vi "WriteDB.vi"(1 "NG?":bool, 4 "曲线数组":refnum<vi>[](array[refnum])) -> ()   [LabVIEW 2018]
uses:
  <vilib>/addons/database/Connection.llb/DB Tools Open Connec (Path).vi
  <vilib>/addons/database/NI_Database_API.lvlib
panel:
  in  "停止":bool
  out "上传状态":string
  in  "SQL_Data":T1={"cMacCode"="1-C-229", "cInvCode"="F100151288", "cCheckDate"="2018-10-31 13:02:50", "cCheckNo"="00013", "cState"="OK", "cDefine1"="OK", "cDefine2"="OK", "cDefine3"="OK", "cDefine4"="OK", "cDefine5"="OK", "cDefine6"="OK", "cDefine7"="8.78", "cDefine8"="6.96", "cDefine9"="2.24", "cDefine10"="1.64", "cDefine11"="1.74", "cDefine12"="+0.54", "cDefine13"="1.48", "cDefine14"="1.47", "cDefine15"="2.07", "cDefine16"="+0.51", "cDefine17"="0", "cDefine18"="0", "cDefine20"="0", "cDefine19"="0", "cDefine21"="0", "cDefine22"="0", "cDefine23"="0", "cDefine24"="0", "cDefine25"="0", "cDefine26"="0", "cDefine27"="0", "cDefine28"="0", "cDefine29"="0", "cDefine30"="0", "cDefine31"="0", "cDefine32"="0", "cDefine33"="0", "cDefine34"="0", "cDefine35"="0", "cDefine36"="0", "cDefine37"="0", "cDefine38"="0", "cDefine39"="0", "cDefine40"="0", "cDefine41"="0", "cDefine42"="0", "cDefine43"="0", "cDefine44"="0", "cDefine45"="0", "cDefine46"="0", "cDefine47"="0", "cDefine48"="0"} caption="上传数据"
  out "error out":errorcluster caption="错误信息" {"code" format="%.0x"}
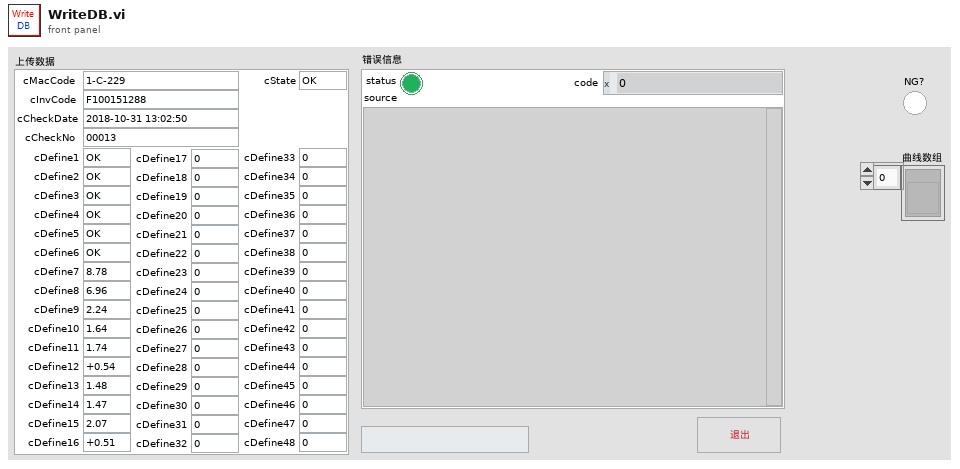
[diagram p1: front panel]
types:
  T1 = cluster{"cMacCode":string, "cInvCode":string, "cCheckDate":string, "cCheckNo":string, "cState":string, "cDefine1":string, "cDefine2":string, "cDefine3":string, "cDefine4":string, "cDefine5":string, "cDefine6":string, "cDefine7":string, "cDefine8":string, "cDefine9":string, "cDefine10":string, "cDefine11":string, "cDefine12":string, "cDefine13":string, "cDefine14":string, "cDefine15":string, "cDefine16":string, "cDefine17":string, "cDefine18":string, "cDefine20":string, "cDefine19":string, "cDefine21":string, "cDefine22":string, "cDefine23":string, "cDefine24":string, "cDefine25":string, "cDefine26":string, "cDefine27":string, "cDefine28":string, "cDefine29":string, "cDefine30":string, "cDefine31":string, "cDefine32":string, "cDefine33":string, "cDefine34":string, "cDefine35":string, "cDefine36":string, "cDefine37":string, "cDefine38":string, "cDefine39":string, "cDefine40":string, "cDefine41":string, "cDefine42":string, "cDefine43":string, "cDefine44":string, "cDefine45":string, "cDefine46":string, "cDefine47":string, "cDefine48":string}
  T2 = typedef "NI_Database_API.lvlib/Conn ObjectReference.ctl" = refnum<k1>
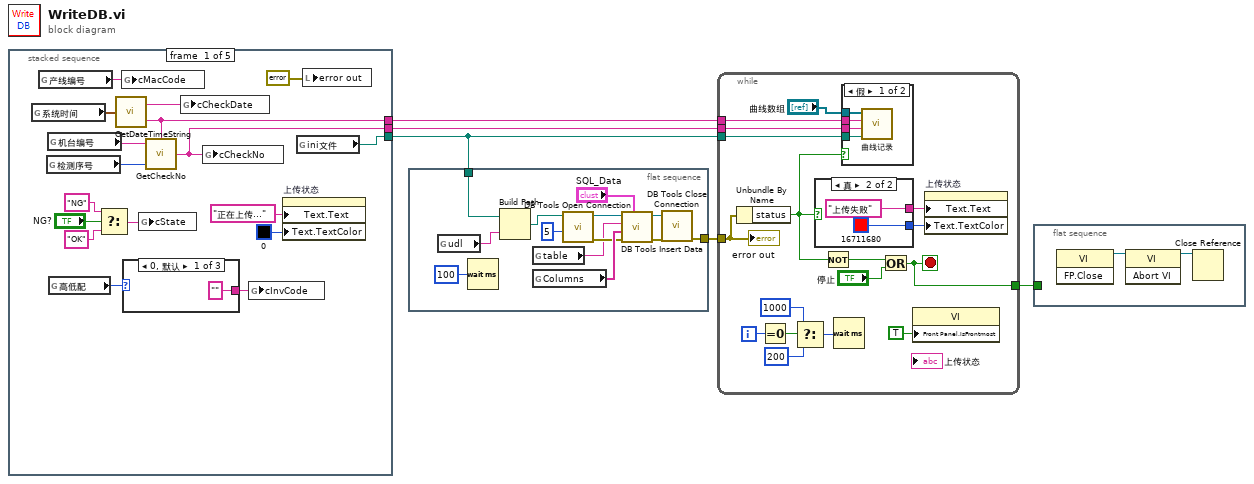
[diagram p0: block diagram]
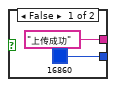
[diagram p3: hidden frame]
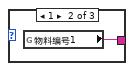
[diagram p4: hidden frame]
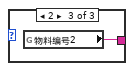
[diagram p5: hidden frame]
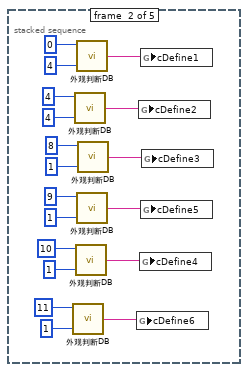
[diagram p6: hidden frame]
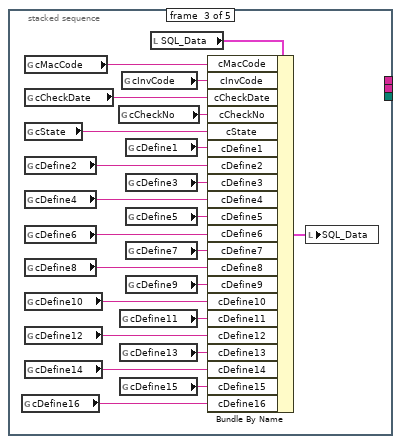
[diagram p7: hidden frame]
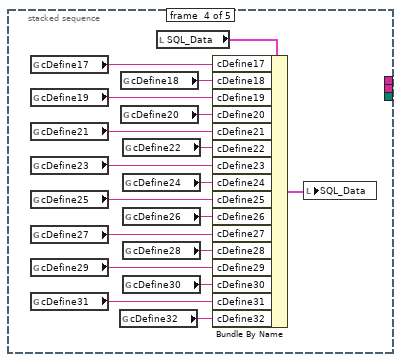
[diagram p8: hidden frame]
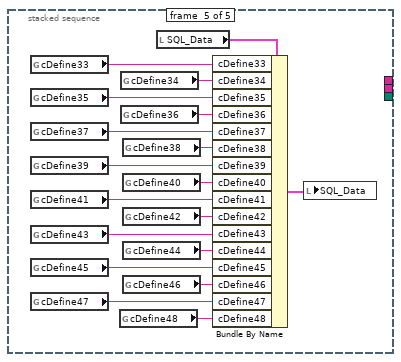
[diagram p9: hidden frame]
diagram:
  n1 = stacked-sequence {
    tunnel: [w8 _ _ _ _] -> w2
    tunnel: [w7 _ _ _ _] -> w3
    tunnel: [w6 _ _ _ _] -> w1
    frame #0 {
      n2 = global read "全局 1.vi" "系统时间"() -> (w9:timestamp)
      n3 = global read "全局 1.vi" "产线编号"() -> (w20:string)
      n4 = global read "全局 1.vi" "检测序号"() -> (w17:u16)
      n5 = global read "全局 1.vi" "机台编号"() -> (w18:string)
      n6 = global read "全局 1.vi" "高低配"() -> (w22:i16)
      n7 = Select(t="NG", s="NG?", f="OK") -> (s? t:f=w12:string)
      n8 = call "GetDateTimeString.vi"("time stamp"=w9) -> ("YYYYMMDD"=w7:string, "date/time string"=w19:string)  [unwired: 3 in]
      n9 = global write "全局SQL.vi" "cMacCode"(w20) -> ()
      n10 = case shown="0, 默认" w22 {
        tunnel: ["" ("物料编号2") w24 w25] -> w21
        frame 0, Default {
        }
        frame 1 {
          n11 = global read "全局 1.vi" "物料编号1"() -> (w24:string)
        }
        frame 2 {
          n12 = global read "全局 1.vi" "物料编号2"() -> (w25:string)
        }
      }
      n13 = global write "全局SQL.vi" "cState"(w12) -> ()
      n14 = call "GetCheckNo.vi"("年月日"=w7, "序号"=w17, "机台编号"=w18) -> ("CheckNo"=w8:string)  [unwired: 1 in]
      n15 = global write "全局SQL.vi" "cCheckDate"(w19) -> ()
      n16 = global write "全局SQL.vi" "cCheckNo"(w8) -> ()
      n17 = global write "全局SQL.vi" "cInvCode"(w21) -> ()
      n18 = property on="上传状态" class="Str"("Text.Text"="正在上传..." ("上传状态"), "Text.TextColor"=u32 0) -> ()  [unwired: 2 in, 2 out]
      n19 = global read "全局 1.vi" "ini文件"() -> (w6:path)
      n20 = local write "error out"(errorcluster {"status"=FALSE, "code"=0, "source"=""} ("错误常量")) -> ()
    }
    frame #1 {
      n21 = call "外观判断DB.vi"("点数"=1 ("长度"), "起点"=11 ("索引")) -> ("结果"=w27:string)  [unwired: 2 in]
      n22 = call "外观判断DB.vi"("点数"=4 ("长度"), "起点"=4 ("索引")) -> ("结果"=w38:string)  [unwired: 2 in]
      n23 = call "外观判断DB.vi"("点数"=1 ("长度"), "起点"=10 ("索引")) -> ("结果"=w30:string)  [unwired: 2 in]
      n24 = call "外观判断DB.vi"("点数"=4 ("长度"), "起点"=0 ("索引")) -> ("结果"=w41:string)  [unwired: 2 in]
      n25 = call "外观判断DB.vi"("点数"=1 ("长度"), "起点"=9 ("索引")) -> ("结果"=w33:string)  [unwired: 2 in]
      n26 = call "外观判断DB.vi"("点数"=1 ("长度"), "起点"=8 ("索引")) -> ("结果"=w36:string)  [unwired: 2 in]
      n27 = global write "全局SQL.vi" "cDefine6"(w27) -> ()
      n28 = global write "全局SQL.vi" "cDefine2"(w38) -> ()
      n29 = global write "全局SQL.vi" "cDefine4"(w30) -> ()
      n30 = global write "全局SQL.vi" "cDefine1"(w41) -> ()
      n31 = global write "全局SQL.vi" "cDefine5"(w33) -> ()
      n32 = global write "全局SQL.vi" "cDefine3"(w36) -> ()
    }
    frame #2 {
      n33 = global read "全局SQL.vi" "cDefine16"() -> (w48:string)
      n34 = global read "全局SQL.vi" "cMacCode"() -> (w66:string)
      n35 = global read "全局SQL.vi" "cCheckDate"() -> (w47:string)
      n36 = global read "全局SQL.vi" "cState"() -> (w64:string)
      n37 = global read "全局SQL.vi" "cDefine2"() -> (w62:string)
      n38 = global read "全局SQL.vi" "cDefine4"() -> (w60:string)
      n39 = global read "全局SQL.vi" "cDefine6"() -> (w58:string)
      n40 = global read "全局SQL.vi" "cDefine8"() -> (w56:string)
      n41 = global read "全局SQL.vi" "cDefine10"() -> (w54:string)
      n42 = global read "全局SQL.vi" "cDefine12"() -> (w52:string)
      n43 = global read "全局SQL.vi" "cDefine14"() -> (w50:string)
      n44 = global read "全局SQL.vi" "cCheckNo"() -> (w46:string)
      n45 = global read "全局SQL.vi" "cDefine11"() -> (w53:string)
      n46 = global read "全局SQL.vi" "cDefine13"() -> (w51:string)
      n47 = global read "全局SQL.vi" "cDefine15"() -> (w49:string)
      n48 = global read "全局SQL.vi" "cInvCode"() -> (w65:string)
      n49 = global read "全局SQL.vi" "cDefine1"() -> (w63:string)
      n50 = global read "全局SQL.vi" "cDefine3"() -> (w61:string)
      n51 = global read "全局SQL.vi" "cDefine5"() -> (w59:string)
      n52 = global read "全局SQL.vi" "cDefine7"() -> (w57:string)
      n53 = global read "全局SQL.vi" "cDefine9"() -> (w55:string)
      n54 = local read "SQL_Data"() -> (w44:T1)
      n55 = Bundle By Name(cluster=w44, "cMacCode"=w66, "cInvCode"=w65, "cCheckDate"=w47, "cCheckNo"=w46, "cState"=w64, "cDefine1"=w63, "cDefine2"=w62, "cDefine3"=w61, "cDefine4"=w60, "cDefine5"=w59, "cDefine6"=w58, "cDefine7"=w57, "cDefine8"=w56, "cDefine9"=w55, "cDefine10"=w54, "cDefine11"=w53, "cDefine12"=w52, "cDefine13"=w51, "cDefine14"=w50, "cDefine15"=w49, "cDefine16"=w48) -> (w45:T1)
      n56 = local write "SQL_Data"(w45) -> ()
    }
    frame #3 {
      n57 = global read "全局SQL.vi" "cDefine17"() -> (w84:string)
      n58 = global read "全局SQL.vi" "cDefine19"() -> (w70:string)
      n59 = global read "全局SQL.vi" "cDefine21"() -> (w82:string)
      n60 = global read "全局SQL.vi" "cDefine23"() -> (w80:string)
      n61 = global read "全局SQL.vi" "cDefine25"() -> (w78:string)
      n62 = global read "全局SQL.vi" "cDefine27"() -> (w76:string)
      n63 = global read "全局SQL.vi" "cDefine29"() -> (w74:string)
      n64 = global read "全局SQL.vi" "cDefine31"() -> (w72:string)
      n65 = global read "全局SQL.vi" "cDefine32"() -> (w71:string)
      n66 = global read "全局SQL.vi" "cDefine18"() -> (w83:string)
      n67 = global read "全局SQL.vi" "cDefine20"() -> (w69:string)
      n68 = global read "全局SQL.vi" "cDefine22"() -> (w81:string)
      n69 = global read "全局SQL.vi" "cDefine24"() -> (w79:string)
      n70 = global read "全局SQL.vi" "cDefine26"() -> (w77:string)
      n71 = global read "全局SQL.vi" "cDefine28"() -> (w75:string)
      n72 = global read "全局SQL.vi" "cDefine30"() -> (w73:string)
      n73 = local read "SQL_Data"() -> (w68:T1)
      n74 = Bundle By Name(cluster=w68, "cDefine17"=w84, "cDefine18"=w83, "cDefine19"=w70, "cDefine20"=w69, "cDefine21"=w82, "cDefine22"=w81, "cDefine23"=w80, "cDefine24"=w79, "cDefine25"=w78, "cDefine26"=w77, "cDefine27"=w76, "cDefine28"=w75, "cDefine29"=w74, "cDefine30"=w73, "cDefine31"=w72, "cDefine32"=w71) -> (w67:T1)
      n75 = local write "SQL_Data"(w67) -> ()
    }
    frame #4 {
      n76 = global read "全局SQL.vi" "cDefine33"() -> (w102:string)
      n77 = global read "全局SQL.vi" "cDefine35"() -> (w88:string)
      n78 = global read "全局SQL.vi" "cDefine37"() -> (w100:string)
      n79 = global read "全局SQL.vi" "cDefine39"() -> (w98:string)
      n80 = global read "全局SQL.vi" "cDefine41"() -> (w96:string)
      n81 = global read "全局SQL.vi" "cDefine43"() -> (w94:string)
      n82 = global read "全局SQL.vi" "cDefine45"() -> (w92:string)
      n83 = global read "全局SQL.vi" "cDefine47"() -> (w90:string)
      n84 = global read "全局SQL.vi" "cDefine48"() -> (w89:string)
      n85 = global read "全局SQL.vi" "cDefine34"() -> (w101:string)
      n86 = global read "全局SQL.vi" "cDefine36"() -> (w87:string)
      n87 = global read "全局SQL.vi" "cDefine38"() -> (w99:string)
      n88 = global read "全局SQL.vi" "cDefine40"() -> (w97:string)
      n89 = global read "全局SQL.vi" "cDefine42"() -> (w95:string)
      n90 = global read "全局SQL.vi" "cDefine44"() -> (w93:string)
      n91 = global read "全局SQL.vi" "cDefine46"() -> (w91:string)
      n92 = local read "SQL_Data"() -> (w86:T1)
      n93 = Bundle By Name(cluster=w86, "cDefine33"=w102, "cDefine34"=w101, "cDefine35"=w88, "cDefine36"=w87, "cDefine37"=w100, "cDefine38"=w99, "cDefine39"=w98, "cDefine40"=w97, "cDefine41"=w96, "cDefine42"=w95, "cDefine43"=w94, "cDefine44"=w93, "cDefine45"=w92, "cDefine46"=w91, "cDefine47"=w90, "cDefine48"=w89) -> (w85:T1)
      n94 = local write "SQL_Data"(w85) -> ()
    }
  }
  n95 = flat-sequence {
    tunnel: [w110] -> w5
    tunnel: w1 -> [w103]
    frame #0 {
      n96 = global read "全局SQL.vi" "udl"() -> (w107:string)
      n97 = Wait (ms)(milliseconds to wait=u32 100 ("等待时间（毫秒）")) -> ()  [unwired: 1 out]
      n98 = Build Path(base path=w103, name or relative path=w107) -> (appended path=w109:path)
      n99 = global read "全局SQL.vi" "table"() -> (w106:string)
      n100 = global read "全局SQL.vi" "Columns"() -> (w115:string[])
      n101 = call-poly <vilib>:"DB Tools Open Connection.vi"("connection timeout (15)"=5, "connection information"=w109) -> ("error out"=w113:errorcluster, "connection reference"=w111:T2)  [unwired: 6 in]
      n102 = call <vilib>:"DB Tools Insert Data.vi"("data"="SQL_Data", "error in (no error)"=w113, "columns"=w115, "table"=w106, "connection reference"=w111) -> ("error out"=w114:errorcluster, "connection reference out"=w112:T2)  [unwired: 5 in]
      n103 = call <vilib>:"DB Tools Close Connection.vi"("error in (no error)"=w114, "connection reference"=w112) -> ("error out"=w110:errorcluster)  [unwired: 5 in]
    }
  }
  n104 = while {
    tunnel: w5 -> [w127]
    tunnel: [w120] -> w4
    tunnel: w2 -> [w119]
    tunnel: w3 -> [w118]
    tunnel: w1 -> [w117]
    i -> [w132]
    stop <- w120 stop-if-true
    n105 = Unbundle By Name(w127) -> ("status"=w121:bool)
    n106 = Equal To 0?(x=w132) -> (x = 0?=w131:bool)
    n107 = Select(t=u32 1000 ("等待时间（毫秒）"), s=w131, f=u32 200) -> (s? t:f=w129:u32)
    n108 = case shown="真" w121 {
      tunnel: ["上传成功" "上传失败"] -> w126
      tunnel: [u32 16860 u32 16711680] -> w125
      frame False {
      }
      frame True {
      }
    }
    n109 = Not(x=w121) -> (.not. x?=w123:bool)
    n110 = Wait (ms)(milliseconds to wait=w129) -> ()  [unwired: 1 out]
    n111 = case shown="假" w121 {
      tunnel: "曲线数组" -> [w133 _]
      tunnel: w119 -> [w135 _]
      tunnel: w118 -> [w134 _]
      tunnel: w117 -> [w136 _]
      frame False {
        n112 = call "曲线记录.vi"("基路径"=w136, "检测序号"=w135, "YYYYMMDD"=w134, "曲线数组"=w133) -> ()  [unwired: 8 in]
      }
      frame True {
      }
    }
    n113 = Or(x=w123, y="停止") -> (x .or. y?=w120:bool)
    n114 = property class="VI"("Front Panel.IsFrontmost"=TRUE ("前面板窗口:在最前")) -> ()  [unwired: 2 in, 2 out]
    n115 = property on="上传状态" class="Str"("Text.Text"=w126, "Text.TextColor"=w125) -> ()  [unwired: 2 in, 2 out]
    "error out" <- w127
  }
  n116 = flat-sequence {
    tunnel: w4 -> [_]
    frame #0 {
      n117 = invoke class="VI" method="FP.Close"() -> (reference out=w142:refnum<vi>)  [unwired: 3 in, 2 out]
      n118 = invoke class="VI" method="Abort VI"(reference=w142) -> (reference out=w141:refnum<vi>)  [unwired: 2 in, 2 out]
      n119 = Close Reference(reference=w141) -> ()  [unwired: 1 in, 1 out]
    }
  }
